vi "Project Documentation Tool.vi"() -> ()   [LabVIEW 2020]
uses:
  <vilib>/regexp/Match Regular Expression.xnode
  LV Project Items Parser.lvlib
panel:
  in  "Close Panel?":bool
  in  "Tree":string(tree)
  out "Selected Item":string
  in  "VI Description":string
  out "VI Icon":picture
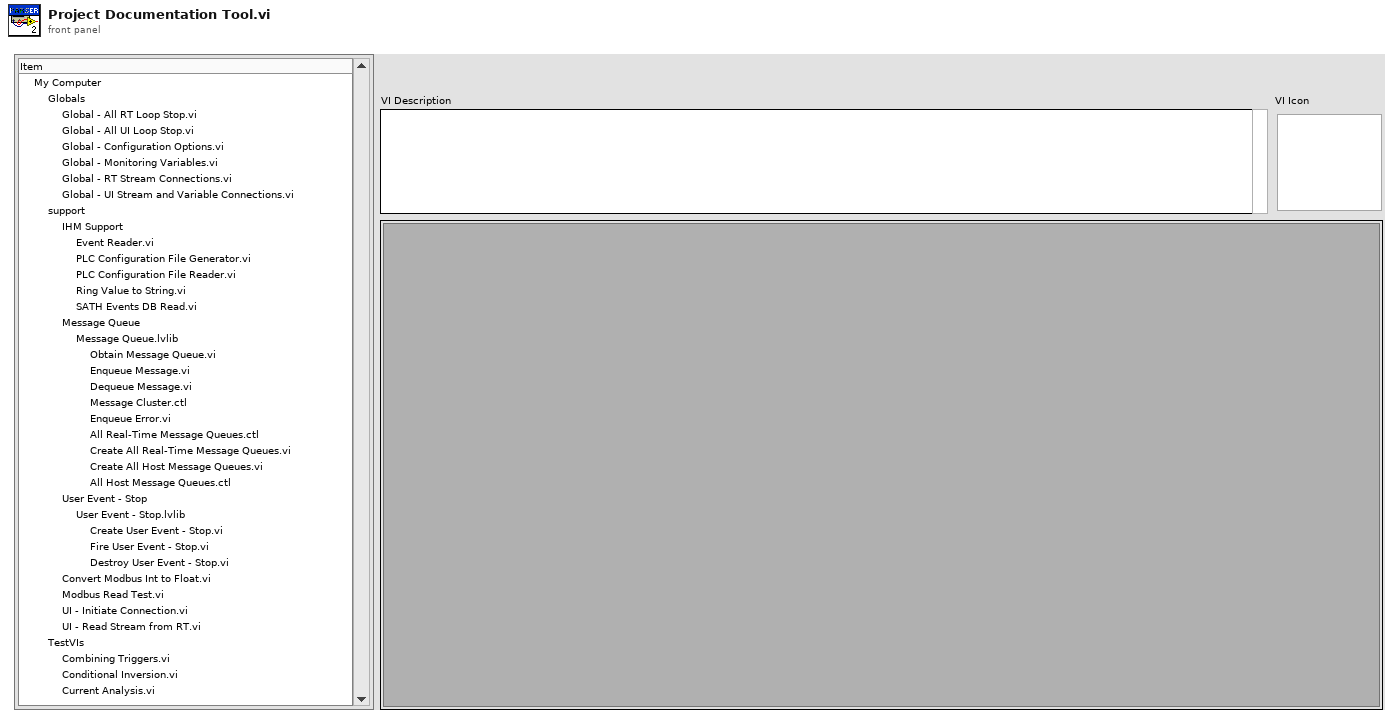
[diagram p1: front panel]
types:
  T1 = enum32{"None", "LabVIEW", "Mac OS", "Windows", "Default"}
  T2 = cluster{"Left Cell String":string, "Child Text":string[], "Child Tag":string, "Item Indent":i32, "Child Only?":bool, "Glyph Index":i32}[]
  T3 = enum32{"Invalid", "Standard", "Closed", "Hidden", "Minimized", "Maximized"}
  T4 = typedef "imagedata.ctl" = cluster{"image type":i32, "image depth":i32, "image":u8[], "mask":u8[], "colors":u32[], "Rectangle":cluster{"left":i16, "top":i16, "right":i16, "bottom":i16}}
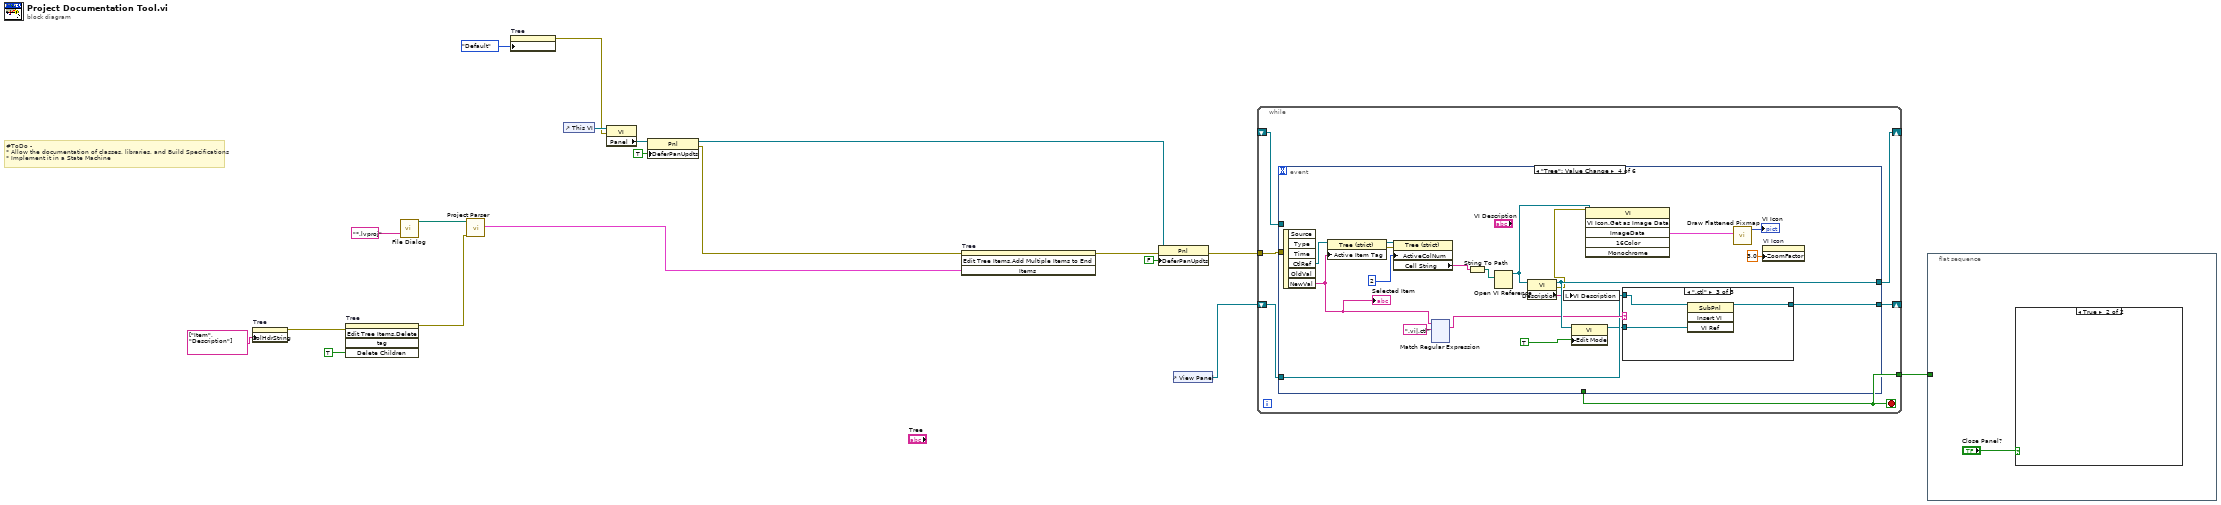
[diagram p0: block diagram]
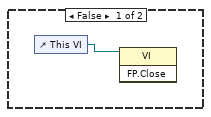
[diagram p2: hidden frame]
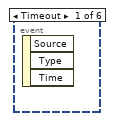
[diagram p3: hidden frame]
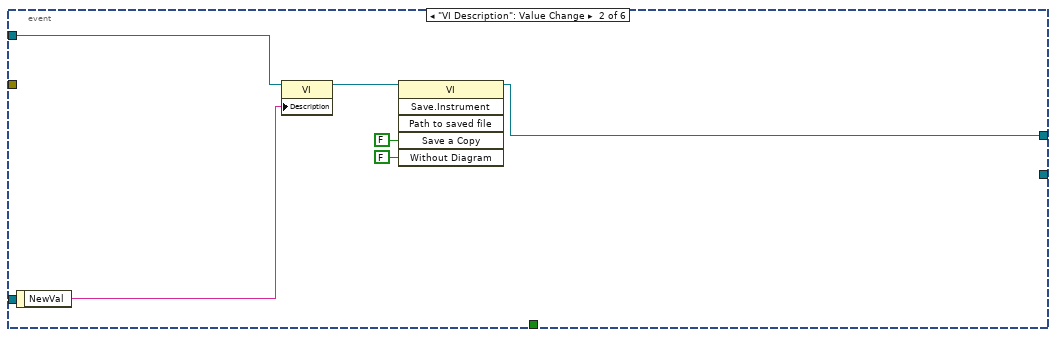
[diagram p4: hidden frame]
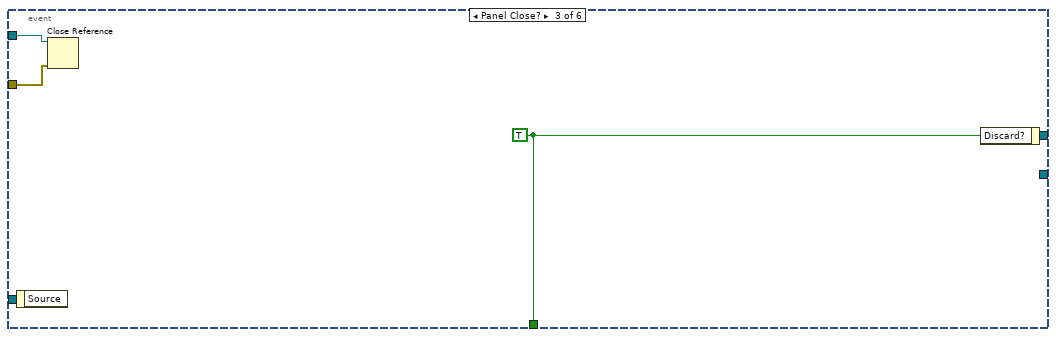
[diagram p5: hidden frame]
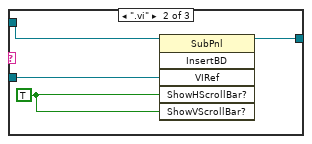
[diagram p7: hidden frame]
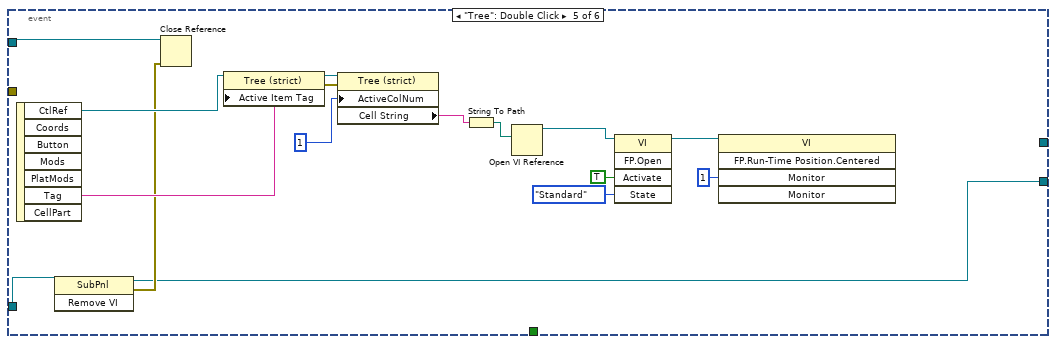
[diagram p8: hidden frame]
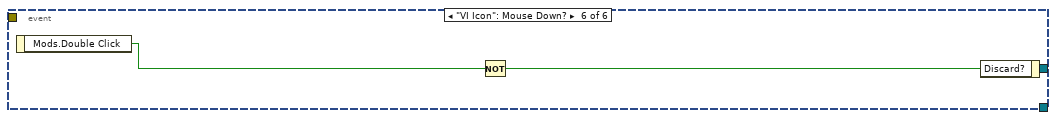
[diagram p9: hidden frame]
diagram:
  # "#ToDo - \n* Allow the documentation of classes, libraries, and Build Specifications\n* Implement it in a State Machine"
  n1 = property on="Tree" class="Tree (strict)"("ColHdrString"=string[] ["Item", "Description"] ("Column Header Strings[]")) -> (error out=w18:errorcluster)  [unwired: 2 in, 1 out]
  n2 = invoke on="Tree" class="Tree (strict)" method="Edit Tree Items.Delete"(error in=w18, "Delete Children"=TRUE ("Delete Children?")) -> (error out=w1:errorcluster)  [unwired: 3 in, 4 out]
  n3 = call "File Dialog"("pattern (all files)"="*.lvproj") -> ("selected path"=w3:path)  [unwired: 11 in, 3 out]
  n4 = call "Project Parser.vi"("error in (no error)"=w1, "file path (use dialog)"=w3) -> ("Item out"=w2:T2)  [unwired: 8 in, 1 out]
  n5 = property on="Tree" class="Tree (strict)"("Expand/Contract Symbol Type"=T1."Default" ("Expand/Contract Symbol:Symbol Type")) -> (error out=w6:errorcluster)  [unwired: 2 in, 1 out]
  n6 = control-ref of="This VI"() -> (w14:refnum<vi>)
  n7 = property class="VI"(reference=w14, error in=w6) -> ("Panel"=w13:refnum<vi>)  [unwired: 2 out]
  n8 = property class="Pnl"(reference=w13, "DeferPanUpdts"=TRUE ("Defer Panel Updates")) -> (reference out=w10:refnum<vi>, error out=w5:errorcluster)  [unwired: 1 in]
  n9 = invoke on="Tree" class="Tree (strict)" method="Edit Tree Items.Add Multiple Items to End"(error in=w5, "Items"=w2) -> (error out=w16:errorcluster)  [unwired: 2 in, 3 out]
  n10 = property class="Pnl"(reference=w10, error in=w16, "DeferPanUpdts"=FALSE ("Defer Panel Updates")) -> (error out=w11:errorcluster)  [unwired: 1 out]
  n11 = control-ref of="View Panel"() -> (w8:refnum<vi>)
  n12 = while {
    tunnel: w11 -> [w25]
    shift-right: [w23] -> _
    shift-left: _ -> [w24]
    tunnel: [w22] -> w15
    shift-right: [w20] -> _
    shift-left: w8 -> [w21]
    stop <- w22 stop-if-true
    n13 = event shown="[3] \"Tree\": Value Change" {
      selector: _ -> [_ _ _ _ _ _]
      dyn-events: _ -> [_ _ _ _ _ _]
      timeout: _ -> [_ _ _ _ _ _]
      tunnel: w25 -> [_ _ w32 _ _ _]
      tunnel: [_ w26 _ w49 _ _] -> w23
      tunnel: w24 -> [_ w31 w33 _ w180 _]
      tunnel: [_ _ w34 _ _ _] -> w22
      tunnel: w21 -> [_ _ _ w46 w179 _]
      tunnel: [_ _ _ w45 w177 _] -> w20
      event Timeout {
        n14 = event-data() -> ()  [unwired: 1 in, 3 out]
      }
      event "VI Description": Value Change {
        n15 = event-data() -> ("NewVal"=w30:string)  [unwired: 1 in]
        n16 = property class="VI"(reference=w31, "Description"=w30) -> (reference out=w29:refnum<vi>)  [unwired: 1 in, 1 out]
        n17 = invoke class="VI" method="Save.Instrument"(reference=w29, "Save a Copy"=FALSE, "Without Diagram"=FALSE) -> (reference out=w26:refnum<vi>)  [unwired: 3 in, 5 out]
      }
      event Panel Close? {
        w34 = TRUE ("Discard?")
        n18 = event-data() -> ()  [unwired: 1 in, 1 out]
        n19 = Close Reference(reference=w33, error in (no error)=w32) -> ()  [unwired: 1 out]
        n20 = event-data("Discard?"=w34) -> ()  [unwired: 1 in, 1 out]
      }
      event "Tree": Value Change {
        n21 = event-data() -> ("CtlRef"=w44:refnum<vi>, "NewVal"=w35:string)  [unwired: 1 in, 4 out]
        "Selected Item" <- w35
        n22 = property class="Tree (strict)"(reference=w44, "Active Item Tag"=w35) -> (reference out=w54:refnum<vi>, error out=w53:errorcluster)  [unwired: 1 in]
        n23 = property class="Tree (strict)"(reference=w54, error in=w53, "ActiveColNum"=2) -> ("Cell String"=w51:string)  [unwired: 2 out]
        n24 = xnode "Match Regular Expression"("input string"=w35, "regular expression"=".vi|.ctl") -> ("whole match"=w47:string)  [unwired: 4 in, 4 out]
        n25 = String To Path(string=w51) -> (path=w50:path)
        n26 = Open VI Reference(vi path=w50) -> (vi reference=w40:refnum<vi>)  [unwired: 5 in, 1 out]
        n27 = property class="VI"(reference=w40) -> (reference out=w49:refnum<vi>, error out=w36:errorcluster, "Description"=w43:string)  [unwired: 1 in]
        n28 = local write "VI Description"(w43) -> ()
        n29 = property class="VI"(reference=w49, "Edit Mode"=TRUE ("Edit Mode On Open")) -> (reference out=w42:refnum<vi>)  [unwired: 1 in, 1 out]
        n30 = invoke class="VI" method="VI Icon.Get as Image Data"(reference=w40, error in=w36) -> ("ImageData"=w39:T4)  [unwired: 4 in, 5 out]
        n31 = case shown="\".ctl\"" w47 {
          tunnel: w42 -> [_ w59 w60]
          tunnel: w46 -> [w55 w57 w62]
          tunnel: [w55 w56 w61] -> w45
          frame "False", Default {
          }
          frame ".vi" {
            w58 = TRUE ("ShowHScrollBar")
            n32 = invoke on="Invoke Node" class="SubPnl" method="InsertBD"(reference=w57, "VIRef"=w59, "ShowHScrollBar?"=w58, "ShowVScrollBar?"=w58) -> (reference out=w56:refnum<vi>)  [unwired: 2 in, 5 out]
          }
          frame ".ctl" {
            n33 = invoke class="SubPnl" method="Insert VI"(reference=w62, "VI Ref"=w60) -> (reference out=w61:refnum<vi>)  [unwired: 2 in, 3 out]
          }
        }
        n34 = call <vilib>:"Draw Flattened Pixmap.vi"("image data"=w39) -> ("new picture"=→"VI Icon":picture)  [unwired: 8 in]
        n35 = property on="VI Icon" class="Pict"("ZoomFactor"=sgl 3.0 ("Zoom Factor")) -> ()  [unwired: 2 in, 2 out]
      }
      event "Tree": Double Click {
        n36 = event-data() -> ("CtlRef"=w187:refnum<vi>, "Tag"=w186:string)  [unwired: 1 in, 5 out]
        n37 = invoke class="SubPnl" method="Remove VI"(reference=w179) -> (reference out=w177:refnum<vi>, error out=w178:errorcluster)  [unwired: 2 in, 1 out]
        n38 = Close Reference(reference=w180, error in (no error)=w178) -> ()  [unwired: 1 out]
        n39 = property class="Tree (strict)"(reference=w187, "Active Item Tag"=w186) -> (reference out=w192:refnum<vi>, error out=w191:errorcluster)  [unwired: 1 in]
        n40 = property class="Tree (strict)"(reference=w192, error in=w191, "ActiveColNum"=1) -> ("Cell String"=w189:string)  [unwired: 2 out]
        n41 = String To Path(string=w189) -> (path=w188:path)
        n42 = Open VI Reference(vi path=w188) -> (vi reference=w185:refnum<vi>)  [unwired: 5 in, 1 out]
        n43 = invoke class="VI" method="FP.Open"(reference=w185, "Activate"=TRUE ("Activate?"), "State"=T3."Standard") -> (reference out=w182:refnum<vi>)  [unwired: 2 in, 4 out]
        n44 = invoke class="VI" method="FP.Run-Time Position.Centered"(reference=w182, "Monitor"=i16 1) -> ()  [unwired: 3 in, 5 out]
      }
      event "VI Icon": Mouse Down? {
        n45 = event-data() -> ("Mods.Double Click"=w194:bool)  [unwired: 1 in]
        n46 = Not(x=w194) -> (.not. x?=w193:bool)
        n47 = event-data("Discard?"=w193) -> ()  [unwired: 1 in, 1 out]
      }
    }
  }
  n48 = flat-sequence {
    tunnel: w15 -> [_]
    frame #0 {
      n49 = case shown="True" "Close Panel?" {
        frame False {
          n50 = control-ref of="This VI"() -> (w196:refnum<vi>)
          n51 = invoke class="VI" method="FP.Close"(reference=w196) -> ()  [unwired: 2 in, 3 out]
        }
        frame True {
        }
      }
    }
  }
